vi "Digitizer Strain Configure Quarter Bridge.vi"(0 "instrument handle":refnum<k15>, 1 "InputType (Differential)":i32(ring) items=["Differential", "Sended"], 2 "Mode (Time)":i32(ring) items=["Time", "Frequency"], 3 "SampRate":dbl, 5 "GaugeFactor":dbl, 7 "ExcitationVoltage":dbl, 9 "Range":dbl, 11 "error in (no error)":errorcluster {"code" format="%.0x"}, 12 "Coupling (DC)":i32(ring) items=["DC", "AC"], 13 "SampCount":i32 format="%.0g", 14 "ChannelList":string) -> (4 "instrument handle out":refnum<k15>, 15 "error out":errorcluster {"code" format="%.0x"})   [LabVIEW 2020, in "Keysight DAQ970.lvlib"]
doc: "Configures the specified channels for quarter bridge strain gauge module digitizing, but they do not initiate the digitizing."
uses:
  Keysight DAQ970.lvlib
  KtDAQ970.dll
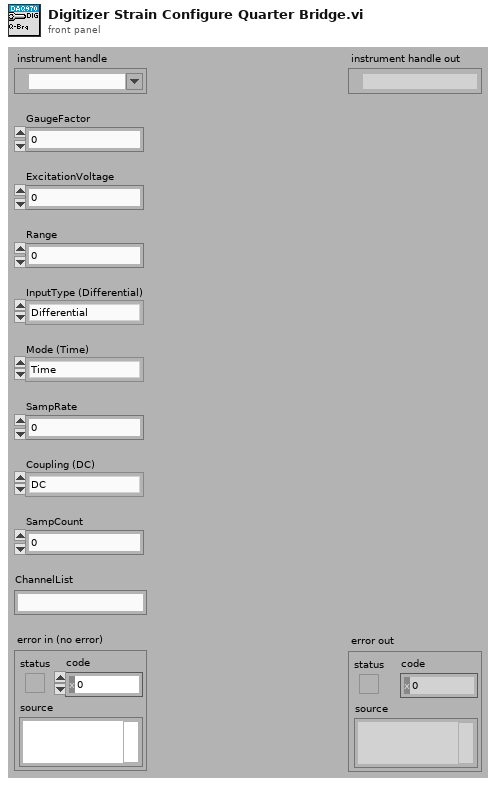
[diagram p1: front panel]
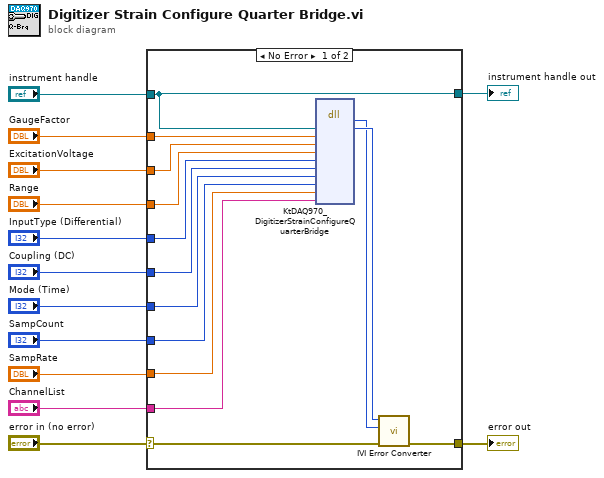
[diagram p0: block diagram]
diagram:
  n1 = case shown="No Error" "error in (no error)" {
    selector: "error in (no error)" -> [w25 w29]
    tunnel: [w24 w29] -> w13
    tunnel: "instrument handle" -> [w14 w28]
    tunnel: "GaugeFactor" -> [w23 _]
    tunnel: "ExcitationVoltage" -> [w22 _]
    tunnel: "Range" -> [w21 _]
    tunnel: "InputType (Differential)" -> [w20 _]
    tunnel: "Coupling (DC)" -> [w19 _]
    tunnel: "Mode (Time)" -> [w18 _]
    tunnel: "SampCount" -> [w17 _]
    tunnel: "SampRate" -> [w16 _]
    tunnel: "ChannelList" -> [w15 _]
    tunnel: [w14 w28] -> w1
    frame No Error {
      n2 = dll-call lib="KtDAQ970**.dll" fn="KtDAQ970_DigitizerStrainConfigureQuarterBridge"("Vi"=w14, "GaugeFactor"=w23, "ExcitationVoltage"=w22, "Range"=w21, "InputType"=w20, "Coupling"=w19, "Mode"=w18, "SampCount"=w17, "SampRate"=w16, "ChannelList"=w15) -> (w26:i32, "Vi"=w27:u32)  [unwired: 12 in, 2 out]
      n3 = call "IVI Error Converter.vi"("error in (no error)"=w25, "IVI error code (0)"=w26, "instrument handle"=w27) -> ("error out"=w24:errorcluster)  [unwired: 7 in, 1 out]
    }
    frame Error {
    }
  }
  "error out" <- w13
  "instrument handle out" <- w1
